vi "group Sync Write Change Param.vi"(6 "data_pos":u16, 7 "data_length":u16, 8 "error in (no error)":errorcluster, 9 "data":u32, 10 "id":u8, 11 "group_num":i32) -> (0 "error out":errorcluster, 3 "function return":u8)   [LabVIEW 2022 SP3, in "dxl.lvlib"]
doc: "WINDECLSPEC uint8_t groupSyncWriteChangeParam (int group_num, uint8_t id, uint32_t data, uint16_t data_length, uint16_t data_pos);"
uses:
  dxl.lvlib
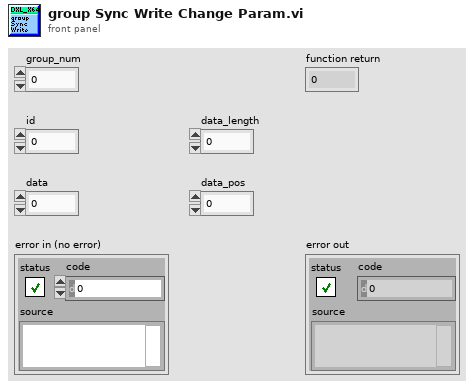
[diagram p1: front panel]
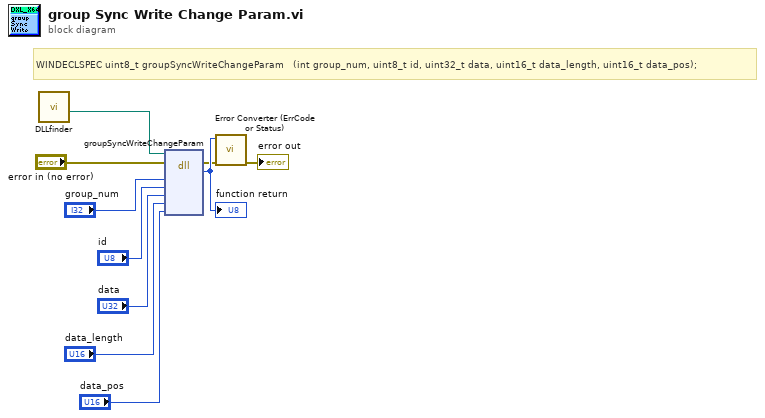
[diagram p0: block diagram]
diagram:
  # "WINDECLSPEC uint8_t groupSyncWriteChangeParam   (int group_num, uint8_t id, uint32_t data, uint16_t data_length, uint16_t data_pos);"
  n1 = call "DLLfinder.vi"() -> ("File Path"=w1:path)  [unwired: 11 in]
  n2 = dll-call lib="C:/EnFlo_Software/ADAM Serial/Instrument drivers/Dynamixel/2nd attempt/Library/dxl_x64_c.*" fn="groupSyncWriteChangeParam"(path in=w1, error in="error in (no error)", "group_num"="group_num", "id"="id", "data"="data", "data_length"="data_length", "data_pos"="data_pos") -> (error out=w3:errorcluster, "return type"=w10:u8)  [unwired: 6 in, 1 out]
  "function return" <- w10
  n3 = call "Error Converter (ErrCode or Status).vi"("error in (no error)"=w3, "error code"=w10) -> ("error out"=→"error out":errorcluster)  [unwired: 9 in]
